vi "Cluster to Array of VData.vi"(8 "error in (no error)":errorcluster, 10 "Cluster":refnum<class "variant.lvclass">) -> (0 "error out":errorcluster, 2 "Array of VData":refnum<class "variant.lvclass">[](array[class]))   [LabVIEW 2020]
doc: "Returns the elements of a cluster as an array of variant data."
uses:
  variant.lvclass
  Type Descriptor/TD.lvclass/TD.ctl
  Bytes/Bytes.lvclass/Bytes.ctl
  Type Descriptor/Cluster/Cluster.lvclass
  Bytes/read.vi
  Bytes/to_data.vi
  Bytes/from_byte_array.vi
  Type Descriptor/TD.lvclass
  C:/projects/OpenG-Variant-Data-Library/source/library/Bytes/Bytes.lvclass
  Bytes/Bytes.lvclass
  <userlib>/_OpenG.lib/error/error.llb/openg_error.lvlib
  C:/projects/OpenG-Variant-Data-Library/source/library/LVData/Type Descriptor/TD.lvclass
  C:/projects/OpenG-Variant-Data-Library/source/library/LVData/Type Descriptor/Cluster/Cluster.lvclass
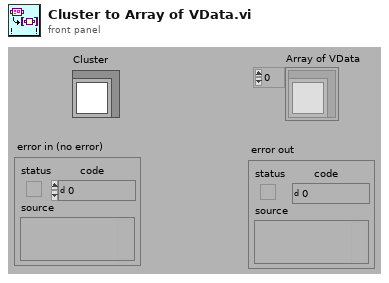
[diagram p1: front panel]
types:
  T1 = typedef "openg_variant.lvlib/Type Descriptor Enumeration.ctl" = enum8{"<Null>", "I8", "I16", "I32", "I64", "U8", "U16", "U32", "U64", "SGL", "DBL", "EXT", "CSG", "CDB", "CXT", "0x0F", "0x10", "0x11", "0x12", "0x13", "0x14", "Enum U8", "Enum U16", "Enum U32", "Enum U64", "SGL PQ", "DBL PQ", "EXT PQ", "CSG PQ", "CDB PQ", "CXT PQ", "0x1F", "0x20", "Boolean", "0x22", "0x23", "0x24", "0x25", "0x26", "0x27", "0x28", "0x29", "0x2A", "0x2B", "0x2C", "0x2D", "0x2E", "0x2F", "String", "0x31", "Path", "Pict", "0x34", "0x35", "0x36", "DAQ", "0x38", "0x39", "0x3A", "0x3B", "0x3C", "0x3D", "0x3E", "0x3F", "Array", "0x41", "0x42", "0x43", "0x44", "0x45", "0x46", "0x47", "0x48", "0x49", "0x4A", "0x4B", "0x4C", "0x4D", "0x4E", "0x4F", "Cluster", "0x51", "0x52", "Variant", "Waveform", "0x55", "0x56", "0x57", "0x58", "0x59", "0x5A", "0x5B", "0x5C", "0x5D", "0x5E", "Fixed Point", "0x60", "0x61", "0x62", "0x63", "0x64", "0x65", "0x66", "0x67", "0x68", "0x69", "0x6A", "0x6B", "0x6C", "0x6D", "0x6E", "0x6F", "Refnum", "0x71", "0x72", "Set Collection", "Map Collection"}
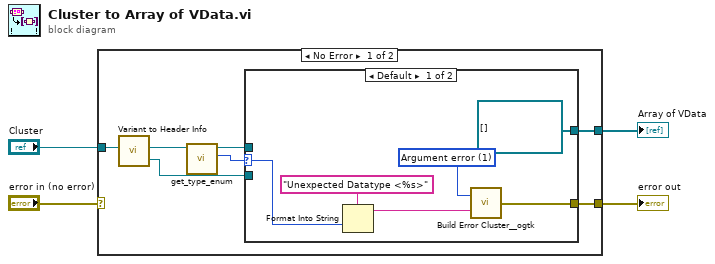
[diagram p0: block diagram]
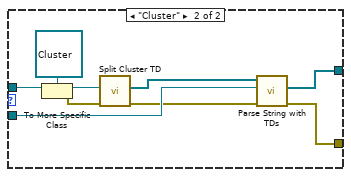
[diagram p2: hidden frame]
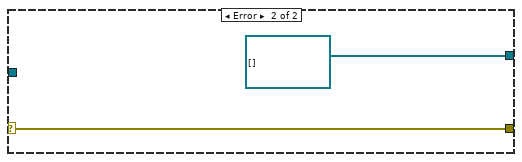
[diagram p3: hidden frame]
diagram:
  n1 = case shown="No Error" "error in (no error)" {
    selector: "error in (no error)" -> [_ w28]
    tunnel: [w11 w28] -> w4
    tunnel: [w10 refnum<class "variant.lvclass">[] [] ("Array of VData")] -> w2
    tunnel: "Cluster" -> [w7 _]
    frame No Error {
      n2 = call "Variant to Header Info.vi"("Variant"=w7) -> ("TypeDescriptor"=w9:refnum<class "TD.lvclass">, "DataString"=w8:refnum<class "DataString.lvclass">)  [unwired: 3 in, 1 out]
      n3 = call "get_type_enum.vi"("TypeDescriptor"=w9) -> ("type"=w5:T1, "TypeDescriptor out"=w6:refnum<class "TD.lvclass">)  [unwired: 9 in]
      n4 = case shown="Default" w5 {
        selector: w5 -> [w14 _]
        tunnel: [w17 w26] -> w11
        tunnel: [refnum<class "variant.lvclass">[] [] ("Array of VData") w25] -> w10
        tunnel: w6 -> [_ w23]
        tunnel: w8 -> [_ w24]
        frame Default {
          w16 = 1 items=["No error", "Argument error", "Memory is full", "Out of zone", "End of file", "File already open", "Generic file I/O error", "File not found", "File permission error", "Disk is full", "Duplicate path", "Too many files open", "System feature not enabled", "Resource file not found", "Cannot add resource", "Resource not found", "Image not found", "Image memory error", "Pen does not exist", "Config type invalid", "Config token not found", "Config parse error", "Config memory error", "Bad external code format", "Bad external code offset", "External code not present", "Null window", "Destroy window error", "Null menu", "Print aborted", "Bad print record", "Print driver error", "Windows error during printing", "Memory error during printing", "Print dialog error", "Generic print error", "Invalid device refnum", "Device not found", "Device parameter error", "Device unit error", "Cannot open device", "Device call aborted", "Generic error", "Cancelled by user", "Object ID too low", "Object ID too high", "Object not in heap", "Unknown heap", "Unknown object (invalid DefProc)", "Unknown object (DefProc not in table)", "Message out of range", "Invalid (null) method", "Unknown message", "Manager call not supported", "Bad address", "Network operation in progress", "Network operation timed out", "Connection is busy", "Network attribute not supported", "Network error", "Address in use", "System out of memory", "Connection aborted", "Connection refused", "Not connected", "Already connected", "Connection closed", "Initialization error (interapplication manager)", "Bad occurrence", "Wait on unbound occurrence handler", "Occurrence queue overflow", "Datalog type conflict", "Unused", "Unrecognized type (interapplication manager)", "Memory corrupt", "Failed to make temporary DLL", "Old CIN version", "Drag socket not found", "Failed to load drop-object", "Failed to register OLE object", "Failed to release OLE object", "Format specifier type mismatch", "Unknown format specifier", "Too few format specifiers", "Too many format specifiers", "Scan failed", "Newer CIN version", "Error converting to variant", "Runtime menu error", "Password tampered", "Variant attribute not found", "Incompatible variant data type", "Event data is not available", "Event Store is not present", "Occurrence is not found", "Event Queue is not created", "Event info is not available", "Refnum passed is NULL", "Error retrieving Class GUID", "Error retrieving CoClass GUID", "Error retrieving TypeLib GUID.", "Bad built application magic bytes.", "Specific driver is different from the specific driver associated with the Logical Name.", "There is no session opened to the class driver.", "Max Error", "MAX - Error with config objects", "MAX - Error loading configuration", "MAX - Group not supported"]
          n5 = Format Into String(format string="Unexpected Datatype <%s>" ("Format String"), w14) -> (resulting string=w13:string)  [unwired: 2 in, 1 out]
          n6 = call <userlib>:"Build Error Cluster__ogtk.vi"("String to Prepend to source (\"\")"=w13, "code"=w16) -> ("error out"=w17:errorcluster)
        }
        frame "Cluster" {
          n7 = To More Specific Class(target class=refnum<class "Cluster.lvclass"> refnum ("ClusterTD"), reference=w23) -> (specific class reference=w20:refnum<class "Cluster.lvclass">, error out=w18:errorcluster)  [unwired: 1 in]
          n8 = call "Split Cluster TD.vi"("error in (no error)"=w18, "Cluster TD"=w20) -> ("error out"=w21:errorcluster, "element TypeDescriptors"=w22:refnum<class "TD.lvclass">[])  [unwired: 8 in]
          n9 = call "Parse String with TDs.vi"("error in (no error)"=w21, "DataString"=w24, "Type Descriptors"=w22) -> ("error out"=w26:errorcluster, "Array of VData"=w25:refnum<class "variant.lvclass">[])  [unwired: 6 in, 1 out]
        }
      }
    }
    frame Error {
    }
  }
  "error out" <- w4
  "Array of VData" <- w2
